vi "rotation_homing.vi"() -> ()   [LabVIEW 2019]
uses:
  <vilib>/DAQmx/write.llb/DAQmx Write (Digital 1D Wfm NChan NSamp).vi
  <vilib>/DAQmx/read.llb/DAQmx Read (Digital Bool 1Line 1Point).vi
  <vilib>/Waveform/DWDTOps.llb/DWDT Digital Size.vi
  global_variables.vi
  <vilib>/DAQmx/create/channels.llb/DAQmx Create Channel (DO-Digital Output).vi
  <vilib>/DAQmx/configure/timing.llb/DAQmx Timing (Sample Clock).vi
  <vilib>/Waveform/DWDTOps.llb/DWDT Uncompress Digital.vi
  <vilib>/DAQmx/miscellaneous.llb/DAQmx Fill In Error Info.vi
  <vilib>/DAQmx/create/channels.llb/DAQmx Create Channel (DI-Digital Input).vi
panel:
  out "switch state":bool=TRUE
  in  "Rotation orientation":bool=TRUE
  in  "Abort movement":bool
  out "duration of movement":dbl=12.0
  in  "pulse duration (T/2)":dbl=0.00036 format="%#_13p"
  in  "pulses to move":i32=15000
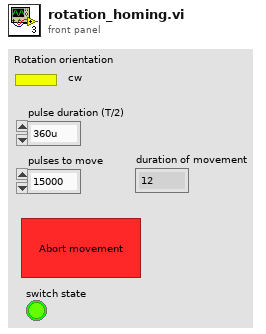
[diagram p1: front panel]
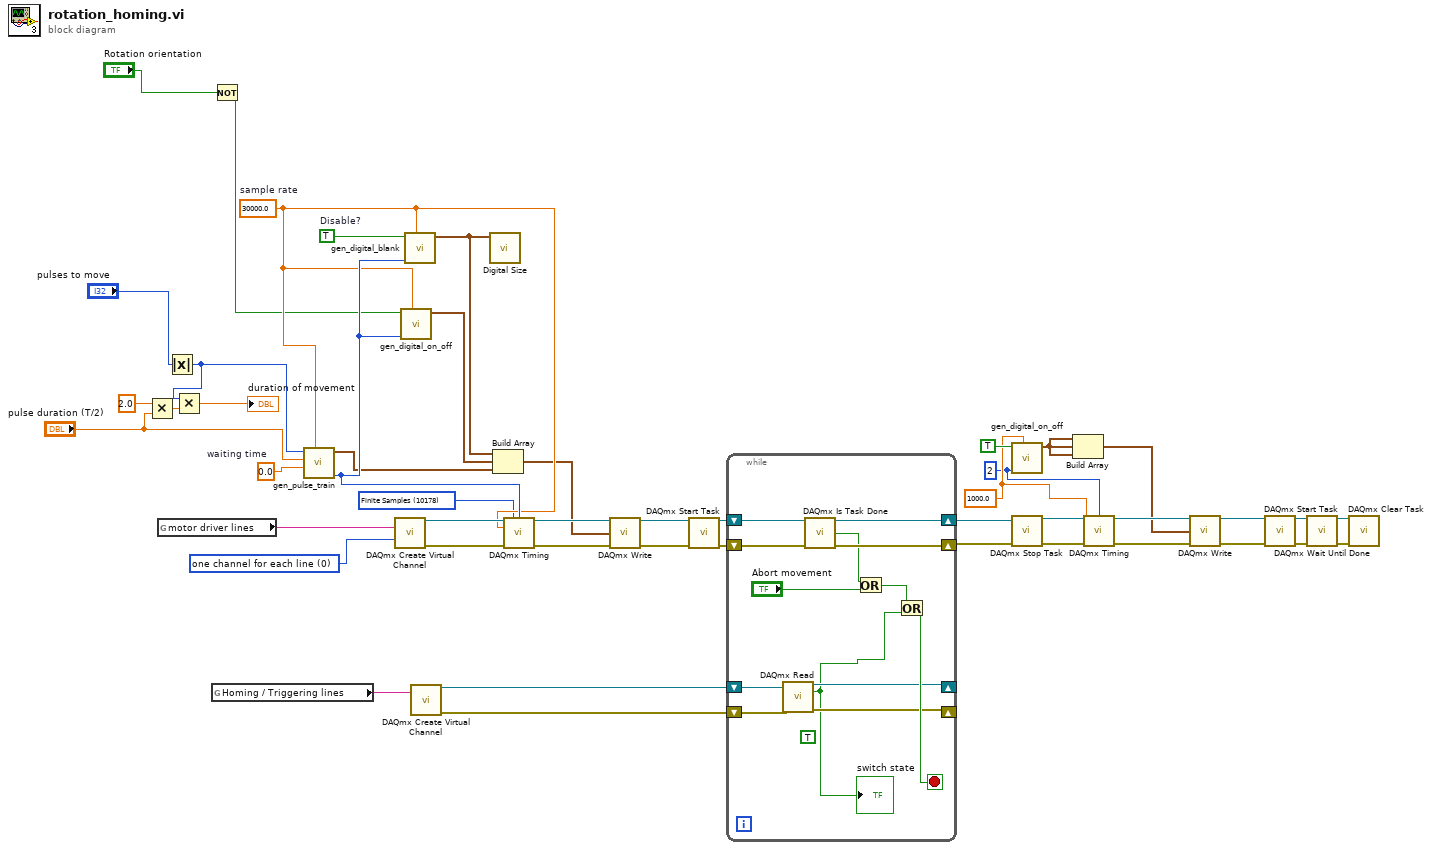
[diagram p0: block diagram]
diagram:
  w9 = 2 ("waveform length")
  w10 = 1000.0 ("rate")
  w33 = 0.0  # waiting time
  w37 = 30000.0  # sample rate
  w36 = TRUE  # Disable?
  w35 = 10178 items=["Finite Samples"=10178, "Continuous Samples"=10123, "Hardware Timed Single Point"=12522] ("sample mode")
  w34 = 0 items=["one channel for each line", "one channel for all lines"] ("line grouping")
  n1 = Multiply(x=2.0, y="pulse duration (T/2)") -> (x*y=w30:dbl)
  n2 = global read "global_variables.vi" "motor driver lines"() -> (w4:tag)
  n3 = Absolute Value(x="pulses to move") -> (abs(x)=w31:i32)
  n4 = Multiply(x=w31, y=w30) -> (x*y=→"duration of movement":dbl)
  n5 = Not(x="Rotation orientation") -> (.not. x?=w1:bool)
  n6 = global read "global_variables.vi" "Homing / Triggering lines"() -> (w3:tag)
  n7 = call "gen_pulse_train.vi"("sampling rate"=w37, "waiting time"=w33, "pulse width"="pulse duration (T/2)", "Number of pulses"=w31) -> ("waveform length"=w44:i32, "digital waveform out"=w42:digitalwaveform)  [unwired: 6 in]
  n8 = call-poly <vilib>:"DAQmx Create Virtual Channel.vi"("lines"=w4, "line grouping"=w34) -> ("task out"=w38:refnum<k21>, "error out"=w41:errorcluster)  [unwired: 12 in]
  n9 = call "gen_digital_on_off.vi"("sampling rate"=w37, "waveform length"=w44, "On / Off"=w1) -> ("digital waveform"=w43:digitalwaveform)  [unwired: 8 in]
  n10 = call "gen_digital_blank.vi"("sampling rate"=w37, "waveform length"=w44, "On / Off"=w36) -> ("digital waveform"=w47:digitalwaveform)  [unwired: 8 in]
  n11 = call-poly <vilib>:"DAQmx Create Virtual Channel.vi"("lines"=w3) -> ("task out"=w7:refnum<k21>, "error out"=w8:errorcluster)  [unwired: 13 in]
  n12 = call-poly <vilib>:"Digital Size.vi"("digital waveform in"=w47) -> ()  [unwired: 7 in, 4 out]
  n13 = Build Array(w47, w43, w42) -> (w6:digitalwaveform[])
  n14 = call-poly <vilib>:"DAQmx Timing.vi"("task/channels in"=w38, "sample mode"=w35, "samples per channel"=w44, "rate"=w37, "error in"=w41) -> ("task out"=w39:refnum<k21>, "error out"=w40:errorcluster)  [unwired: 9 in]
  n15 = call-poly <vilib>:"DAQmx Write.vi"("task/channels in"=w39, "data"=w6, "error in"=w40) -> ("task out"=w45:refnum<k21>, "error out"=w46:errorcluster)  [unwired: 10 in, 1 out]
  n16 = call <vilib>:"DAQmx Start Task.vi"("task/channels in"=w45, "error in"=w46) -> ("task out"=w27:refnum<k21>, "error out"=w26:errorcluster)  [unwired: 12 in]
  n17 = while {
    shift-right: [w57] -> w24
    shift-left: w26 -> [w59]
    shift-right: [w58] -> w25
    shift-left: w27 -> [w60]
    shift-right: [w49] -> _
    shift-left: w7 -> [w52]
    shift-right: [w50] -> _
    shift-left: w8 -> [w51]
    stop <- w53 stop-if-true
    (unwired) TRUE ("Abort movement")
    n18 = call-poly <vilib>:"DAQmx Read.vi"("task/channels in"=w52, "error in"=w51) -> ("task out"=w49:refnum<k21>, "data"=w48:bool, "error out"=w50:errorcluster)  [unwired: 11 in]
    "switch state" <- w48
    n19 = call <vilib>:"DAQmx Is Task Done.vi"("task/channels in"=w60, "error in"=w59) -> ("task out"=w58:refnum<k21>, "task done?"=w55:bool, "error out"=w57:errorcluster)  [unwired: 11 in]
    n20 = Or(x=w55, y="Abort movement") -> (x .or. y?=w54:bool)
    n21 = Or(x=w54, y=w48) -> (x .or. y?=w53:bool)
  }
  n22 = call "gen_digital_on_off.vi"("sampling rate"=w10, "waveform length"=w9, "On / Off"=TRUE) -> ("digital waveform"=w13:digitalwaveform)  [unwired: 8 in]
  n23 = call <vilib>:"DAQmx Stop Task.vi"("task/channels in"=w25, "error in"=w24) -> ("task out"=w14:refnum<k21>, "error out"=w17:errorcluster)  [unwired: 12 in]
  n24 = Build Array(w13, w13, w13) -> (w12:digitalwaveform[])
  n25 = call-poly <vilib>:"DAQmx Timing.vi"("task/channels in"=w14, "samples per channel"=w9, "rate"=w10, "error in"=w17) -> ("task out"=w15:refnum<k21>, "error out"=w16:errorcluster)  [unwired: 10 in]
  n26 = call-poly <vilib>:"DAQmx Write.vi"("task/channels in"=w15, "data"=w12, "error in"=w16) -> ("task out"=w23:refnum<k21>, "error out"=w22:errorcluster)  [unwired: 10 in, 1 out]
  n27 = call <vilib>:"DAQmx Start Task.vi"("task/channels in"=w23, "error in"=w22) -> ("task out"=w21:refnum<k21>, "error out"=w20:errorcluster)  [unwired: 12 in]
  n28 = call <vilib>:"DAQmx Wait Until Done.vi"("task/channels in"=w21, "error in"=w20) -> ("task out"=w19:refnum<k21>, "error out"=w18:errorcluster)  [unwired: 12 in]
  n29 = call <vilib>:"DAQmx Clear Task.vi"("task in"=w19, "error in"=w18) -> ()  [unwired: 13 in, 1 out]
